vi "AIGlobal.vi"() -> ()   [LabVIEW 2025]
panel:
  out "action":i32
  in  "forward":T1(c390)
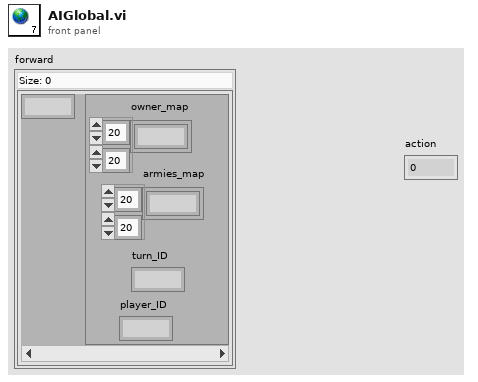
[diagram p1: front panel]
types:
  T1 = map{u32, cluster{"owner_map":i32[][], "armies_map":i32[][], "turn_ID":i32, "player_ID":i32}}
diagram:
